vi "Parse ERDs.vi"(0 "ERD Number":u16 format="%x", 5 "Data":string, 7 "ERD Headers":string[](array[string]), 11 "Error In":errorcluster, 12 "Enable Diagnostic Data":T1) -> (4 "Data":string[][](array[string]), 6 "Length":i32, 15 "Error Out":errorcluster)   [LabVIEW 2016, in "GEA2_Toolkit.lvlib"]
uses:
  library/GEA2_Toolkit.lvlib
  Washer HCC/Washer HCC NEWFI/Type Definitions/HCC Washer Types.ctl
panel:
  out "size(s)":i32[](array[numeric])
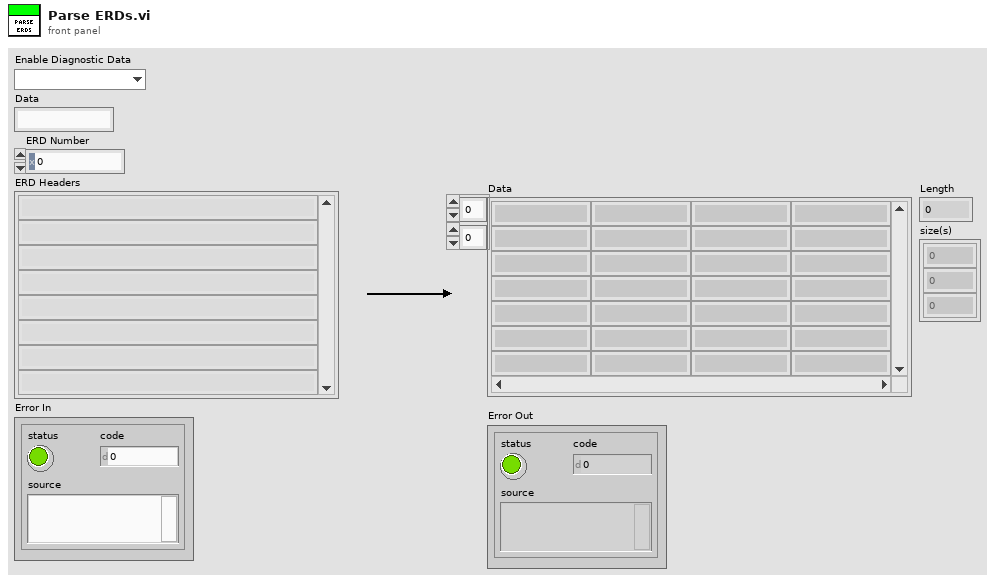
[diagram p1: front panel]
types:
  T1 = typedef "HCC Washer Types.ctl" = enum16{"", "Viper Washer", "Hawk Washer", "2015 Washer", "2017 Washer"}
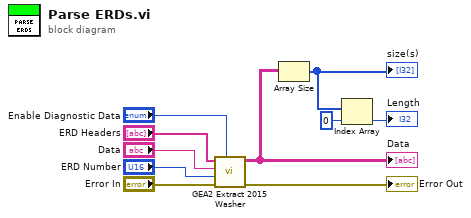
[diagram p0: block diagram]
diagram:
  n1 = call "GEA2 Extract 2015 Washer.vi"("Enable Diagnostic Data"="Enable Diagnostic Data", "Error In"="Error In", "ERD Number"="ERD Number", "Data"="Data", "ERD Headers"="ERD Headers") -> ("Error Out"=→"Error Out":errorcluster, "Array"=w8:string[][])  [unwired: 5 in]
  "Data" <- w8
  n2 = Array Size(array=w8) -> (size(s)=w7:i32[])
  "size(s)" <- w7
  n3 = Index Array(array=w7, index=0) -> (element=→"Length":i32)
